vi "Game整体图.vi"() -> ()   [LabVIEW 2014]
panel:
  in  "Casino":bool
  in  "Backgammon":bool
  in  "Arcade":bool
  in  "Strategy":bool
  in  "Roll":bool
  in  "Reversi":bool
  in  "Moon":bool
  in  "Mines":bool
  in  "Joystick":bool
  in  "Hang man":bool
  in  "Golf":bool
  in  "Games":bool
  in  "Engine":bool
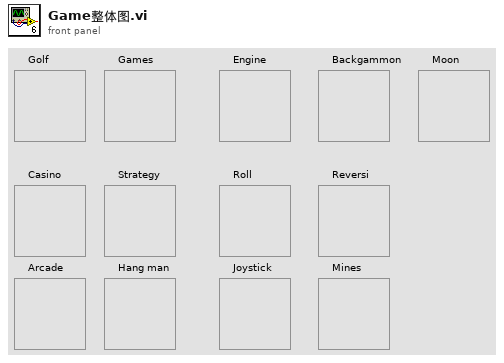
[diagram p1: front panel]
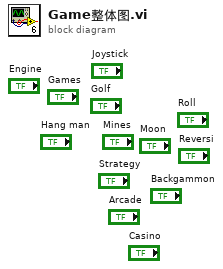
[diagram p0: block diagram]
diagram:
